vi "Agilent 2000 3000 X-Series Acquire Multiple Waveforms.vi"() -> ()   [LabVIEW 2015]
doc: "This example shows how to configure multiple channels and acquire waveforms from multiple channels."
uses:
  <instrlib>/Agilent 2000 3000 X-Series/Agilent 2000 3000 X-Series.lvlib
panel:
  in  "Channel (1: Channel 2)":i32(ring)=1 items=["Channel 1", "Channel 2", "Channel 3", "Channel 4"]
  in  "Channel (0: Channel 1)":i32(ring) items=["Channel 1", "Channel 2", "Channel 3", "Channel 4"]
  in  "Maximum Time (10000 ms)":u32=10000
  in  "Probe Attenuation (1.0)":dbl=1.0
  in  "Vertical Coupling (1: DC)":i32(ring)=1 items=["AC", "DC", "Ground"]
  in  "Probe Attenuation (10.0)":dbl=10.0
  in  "Vertical Coupling (1: DC)":i32(ring)=1 items=["AC", "DC", "Ground"]
  out "Waveform Data":waveform(dbl)[](graph)
  in  "VISA resource name":refnum<visa-resource-name>
  # "(c) 2011-2016 National Instruments.  ALL RIGHTS RESERVED."
  # "Channel A"
  # "Channel B"
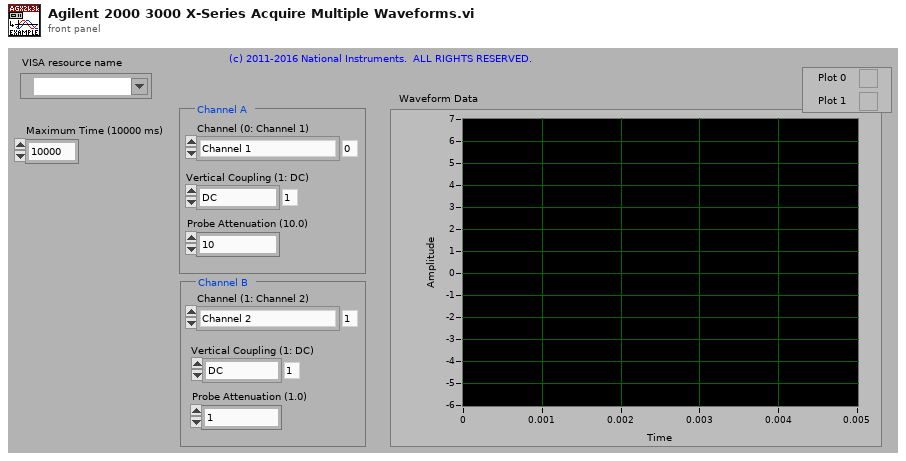
[diagram p1: front panel]
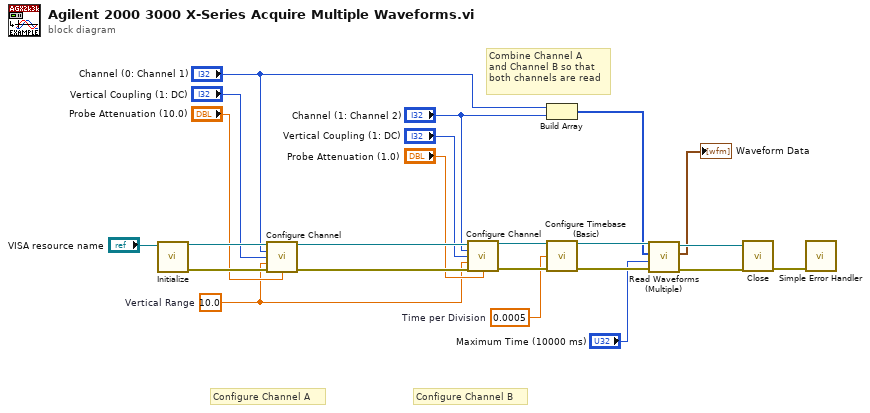
[diagram p0: block diagram]
diagram:
  w4 = 0.0005  # Time per Division
  w7 = 10.0  # Vertical Range
  # "Combine Channel A\nand Channel B so that\nboth channels are read"
  # "Configure Channel B"
  # "Configure Channel A"
  n1 = call <instrlib>:"Initialize.vi"("VISA resource name"="VISA resource name") -> ("error out"=w21:errorcluster, "VISA resource name out"=w20:refnum<visa-resource-name>)  [unwired: 4 in, 5 out]
  n2 = call <instrlib>:"Configure Channel.vi"("VISA resource name"=w20, "Channel Name (0: Channel 1)"="Channel (0: Channel 1)", "Coupling (1: DC)"="Vertical Coupling (1: DC)", "Vertical Range (40.0 V)"=w7, "error in (no error)"=w21, "Probe Attenuation (1.0)"="Probe Attenuation (10.0)") -> ("VISA resource name out"=w19:refnum<visa-resource-name>, "error out"=w18:errorcluster)  [unwired: 5 in, 3 out]
  n3 = call <instrlib>:"Configure Channel.vi"("VISA resource name"=w19, "Channel Name (0: Channel 1)"="Channel (1: Channel 2)", "Coupling (1: DC)"="Vertical Coupling (1: DC)", "Vertical Range (40.0 V)"=w7, "error in (no error)"=w18, "Probe Attenuation (1.0)"="Probe Attenuation (1.0)") -> ("VISA resource name out"=w16:refnum<visa-resource-name>, "error out"=w17:errorcluster)  [unwired: 5 in, 3 out]
  n4 = Build Array("Channel (0: Channel 1)", "Channel (1: Channel 2)") -> (w6:i32[])
  n5 = call <instrlib>:"Configure Timebase (Basic).vi"("VISA resource name"=w16, "Scale (50 s/div)"=w4, "error in (no error)"=w17) -> ("VISA resource name out"=w15:refnum<visa-resource-name>, "error out"=w14:errorcluster)  [unwired: 6 in, 5 out]
  n6 = call <instrlib>:"Read Waveforms (Multiple).vi"("error in (no error)"=w14, "Timeout (10000 ms)"="Maximum Time (10000 ms)", "Channels"=w6, "VISA resource name"=w15) -> ("error out"=w12:errorcluster, "Waveform Data"=→"Waveform Data":waveform(dbl)[], "VISA resource name out"=w13:refnum<visa-resource-name>)  [unwired: 5 out]
  n7 = call <instrlib>:"Close.vi"("error in (no error)"=w12, "VISA resource name"=w13) -> ("error out"=w22:errorcluster)  [unwired: 9 out]
  n8 = call <vilib>:"Simple Error Handler.vi"("error in (no error)"=w22) -> ()  [unwired: 1 in, 8 out]
